vi "BASIC_SUBVI_Mean_sd.vi"(0 "Array":dbl[](array[numeric])) -> (1 "s.d.":dbl, 2 "Mean":dbl, 3 "Array/mean":dbl[](array[numeric]), 4 "Array-mean":dbl[](array[numeric]))   [LabVIEW 2020, in "BasicVIs.lvlib"]
uses:
  BasicVIs.lvlib
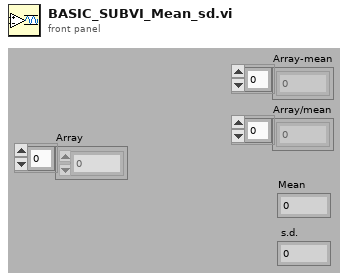
[diagram p1: front panel]
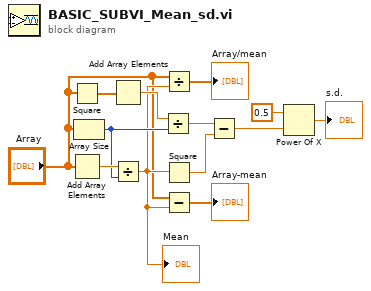
[diagram p0: block diagram]
diagram:
  n1 = Square(x="Array") -> (x^2=w12:dbl[])
  n2 = Add Array Elements(numeric array="Array") -> (sum=w13:dbl)
  n3 = Array Size(array="Array") -> (size(s)=w11:i32)
  n4 = Add Array Elements(numeric array=w12) -> (sum=w10:dbl)
  n5 = Divide(x=w13, y=w11) -> (x/y=w3:dbl)
  "Mean" <- w3
  n6 = Divide(x=w10, y=w11) -> (x/y=w9:dbl)
  n7 = Divide(x="Array", y=w3) -> (x/y=→"Array/mean":dbl[])
  n8 = Square(x=w3) -> (x^2=w8:dbl)
  n9 = Subtract(x="Array", y=w3) -> (x-y=→"Array-mean":dbl[])
  n10 = Subtract(x=w9, y=w8) -> (x-y=w7:dbl)
  n11 = Power Of X(1:w7, 2:0.5 ("y")) -> (0:→"s.d.":dbl)
